vi "simple data display custom vi.vi"(9 "customQueue":refnum<queue>, 11 "parentQueue":refnum<queue>) -> ()   [LabVIEW 2018]
uses:
  custom sub vis/plotControl.ctl
  customViData.ctl
panel:
  out "mainMessage":string caption="Message received from Main VI"
  in  "plotType":bool
  in  "plotControl":T1[](array[typedef])=[{"channel"="time", "X"=TRUE, "Y"=FALSE, "Y2"=FALSE}]
  out "dataTable":string[][](table)
  out "XY Graph":cluster{"New data":dbl[], "New data":dbl[]}[](graph)
  in  "really stop":bool
  in  "quit":bool
  out "ballValve":dbl caption="ball Valve"
  out "butterflyValve":dbl caption="butterfly Valve"
  out "speed":dbl caption="compressor Speed"
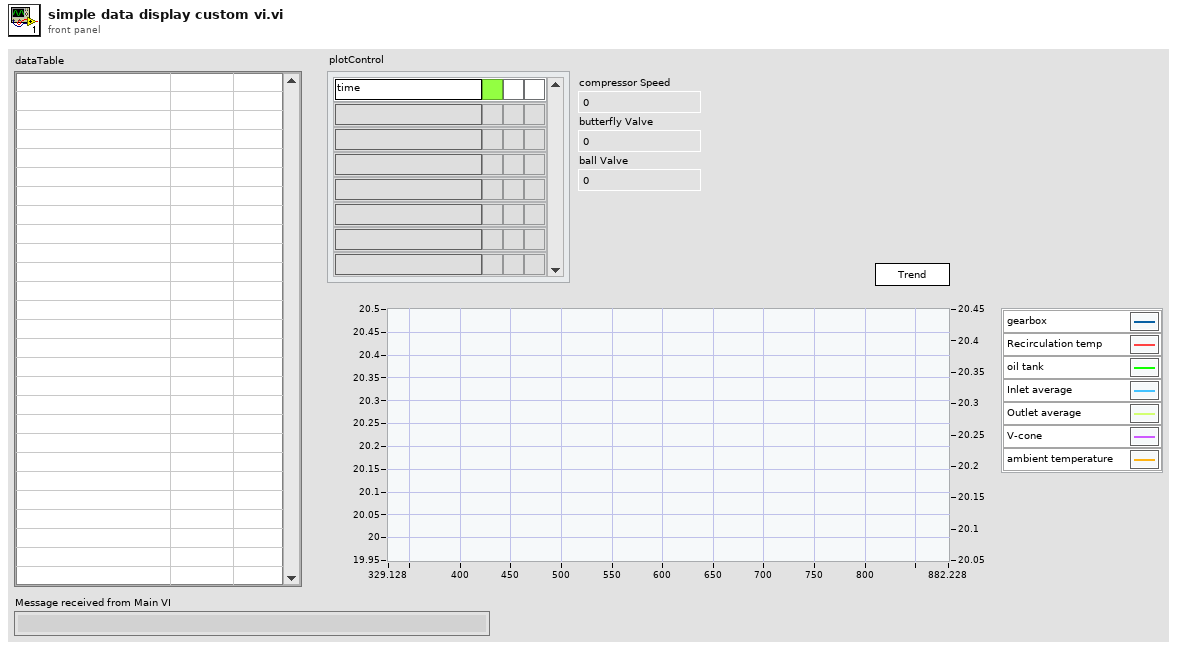
[diagram p1: front panel]
types:
  T1 = typedef "plotControl.ctl" = cluster{"channel":string, "X":bool, "Y":bool, "Y2":bool}
  T2 = typedef "customViData.ctl" = cluster{"rigChannels":string[], "rigUnits":string[], "logging":bool, "plot":cluster{"X":u16[], "Y":u16[], "Y2":u16[]}, "updatePlot":bool, "chartRef":refnum<vi>, "livePlot":bool, "history":dbl[][], "channelCount":i32, "trendIndex":i32}
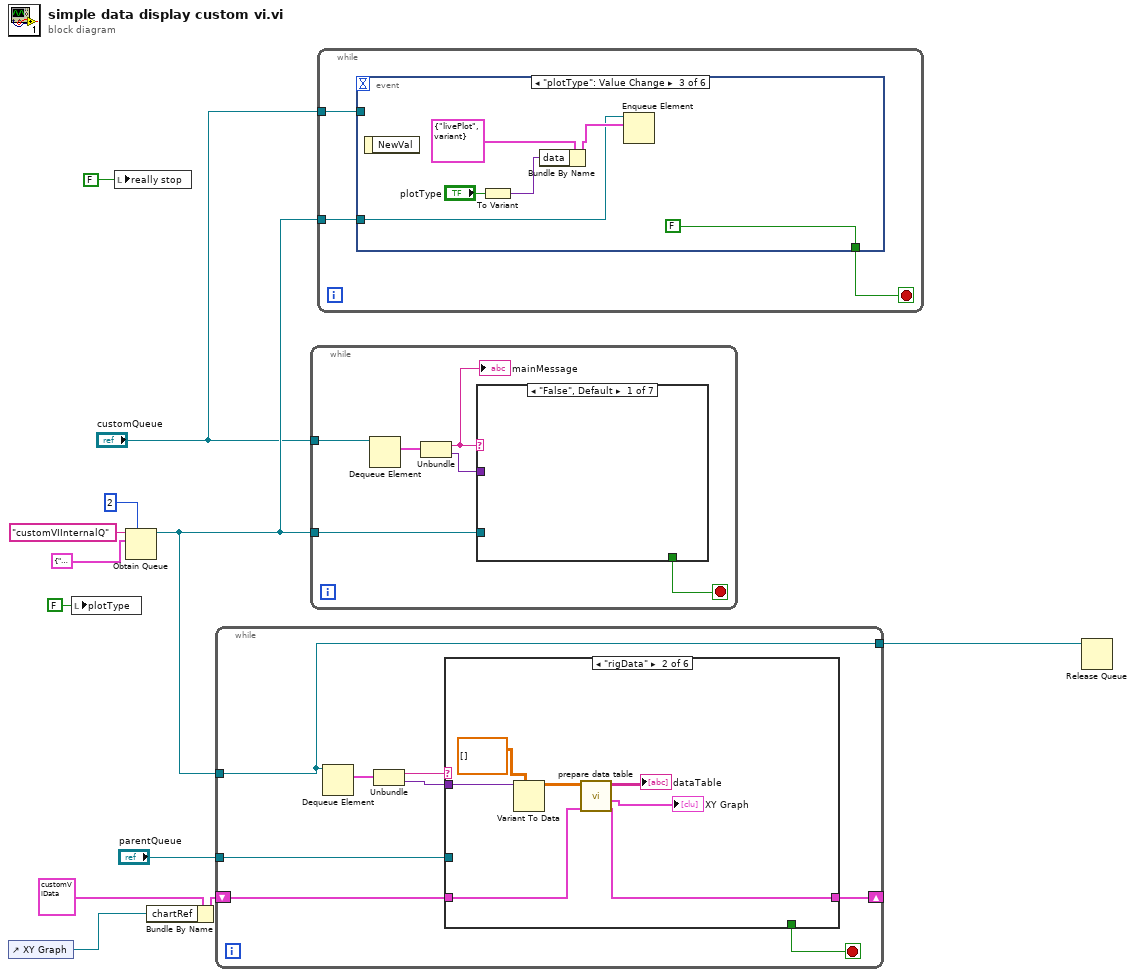
[diagram p0: block diagram]
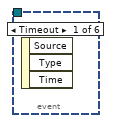
[diagram p2: hidden frame]
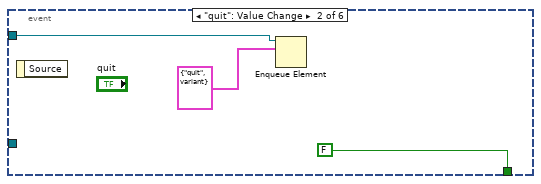
[diagram p3: hidden frame]
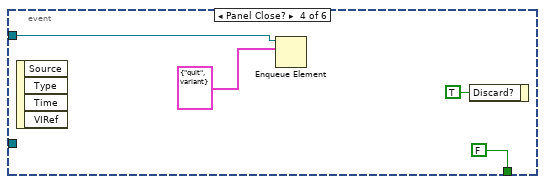
[diagram p4: hidden frame]
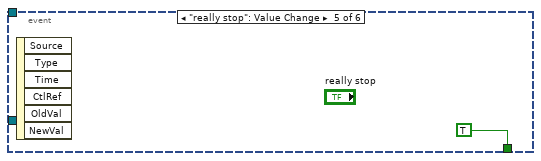
[diagram p5: hidden frame]
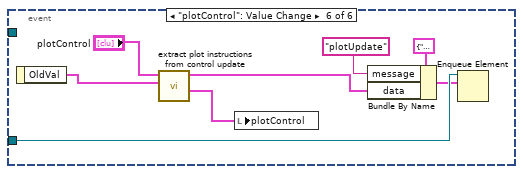
[diagram p6: hidden frame]
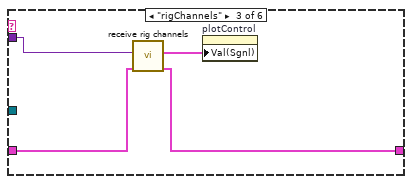
[diagram p8: hidden frame]
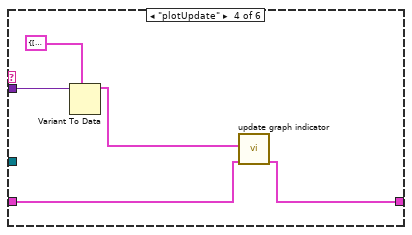
[diagram p9: hidden frame]
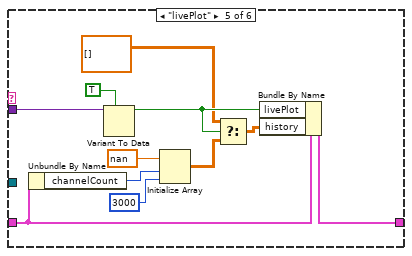
[diagram p10: hidden frame]
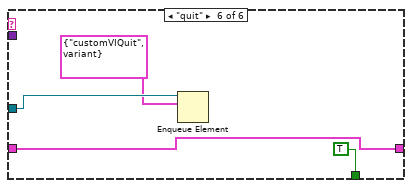
[diagram p11: hidden frame]
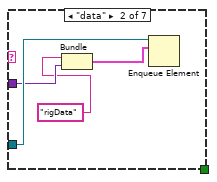
[diagram p12: hidden frame]
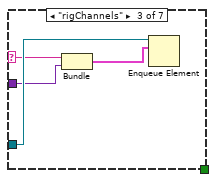
[diagram p13: hidden frame]
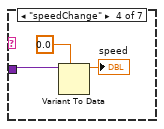
[diagram p14: hidden frame]
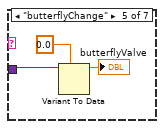
[diagram p15: hidden frame]
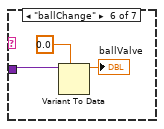
[diagram p16: hidden frame]
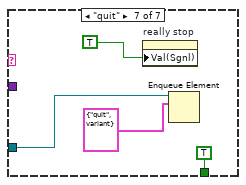
[diagram p17: hidden frame]
diagram:
  n1 = control-ref of="XY Graph"() -> (w2:refnum<vi>)
  n2 = local write "plotType"(FALSE ("plotType")) -> ()
  n3 = local write "really stop"(FALSE) -> ()
  n4 = Obtain Queue(max queue size (-1, unlimited)=2, name (unnamed)="customVIInternalQ", element data type=cluster{"message":string, "data":variant} {"message"="", "data"=variant} ("element")) -> (queue out=w9:refnum<queue>)  [unwired: 2 in, 2 out]
  n5 = Bundle By Name(cluster=T2 {"rigChannels"=[], "rigUnits"=[], "logging"=FALSE, "plot"={"X"=[], "Y"=[], "Y2"=[]}, "updatePlot"=FALSE, "chartRef"=refnum, "livePlot"=FALSE, "history"=[], "channelCount"=0, "trendIndex"=0}, "chartRef"=w2) -> (w3:T2)
  n6 = while {
    tunnel: w9 -> [w15]
    tunnel: "parentQueue" -> [w17]
    tunnel: [w15] -> w7
    shift-right: [w14] -> _
    shift-left: w3 -> [w13]
    stop <- w16 stop-if-true
    n7 = Dequeue Element(queue=w15) -> (element=w20:cluster{"message":string, "data":variant})  [unwired: 2 in, 3 out]
    n8 = Unbundle(w20) -> ("message"=w19:string, "data"=w18:variant)
    n9 = case shown="\"rigData\"" w19 {
      tunnel: w18 -> [_ w28 w32 w37 w47 _]
      tunnel: w17 -> [_ _ _ _ _ w52]
      tunnel: [_ _ _ _ _ TRUE] -> w16
      tunnel: [w21 w23 w30 w34 w48 w49] -> w14
      tunnel: w13 -> [w21 w26 w31 w35 w44 w49]
      frame "", Default {
      }
      frame "rigData" {
        n10 = Variant To Data(type=dbl[][] [], Variant=w28) -> (data=w25:dbl[][])  [unwired: 1 in, 1 out]
        n11 = call "prepare data table.vi"("customViData"=w26, "New data"=w25) -> ("customViData out"=w23:T2, "plot data"=→"XY Graph":cluster{"New data":dbl[], "New data":dbl[]}[], "dataTable"=→"dataTable":string[][])  [unwired: 6 in, 1 out]
      }
      frame "rigChannels" {
        n12 = call "receive rig channels.vi"("customViData in"=w31, "data"=w32) -> ("customViData out"=w30:T2, "updated plotControl"=w29:T1[])  [unwired: 8 in]
        n13 = property on="plotControl" class="Arr (strict)"("Val(Sgnl)"=w29) -> ()  [unwired: 2 in, 2 out]
      }
      frame "plotUpdate" {
        n14 = Variant To Data(type=cluster{"X":u16[], "Y":u16[], "Y2":u16[]} {"X"=[], "Y"=[], "Y2"=[]} ("plot"), Variant=w37) -> (data=w36:cluster{"X":u16[], "Y":u16[], "Y2":u16[]})  [unwired: 1 in, 1 out]
        n15 = call "update graph indicator.vi"("customViData in"=w35, "plot"=w36) -> ("customViData out"=w34:T2)  [unwired: 9 in]
      }
      frame "livePlot" {
        n16 = Unbundle By Name(w44) -> ("channelCount"=w43:i32)
        n17 = Variant To Data(type=TRUE, Variant=w47) -> (data=w41:bool)  [unwired: 1 in, 1 out]
        n18 = Initialize Array(nan ("element"), w43, 3000 ("dimension size")) -> (w39:dbl[][])
        n19 = Select(t=dbl[][] [] ("history"), s=w41, f=w39) -> (s? t:f=w38:dbl[][])
        n20 = Bundle By Name(cluster=w44, "livePlot"=w41, "history"=w38) -> (w48:T2)
      }
      frame "quit" {
        n21 = Enqueue Element(queue=w52, element=cluster{"message":string, "data":variant} {"message"="customVIQuit", "data"=variant}) -> ()  [unwired: 2 in, 3 out]
      }
    }
  }
  n22 = while {
    tunnel: "customQueue" -> [w58]
    tunnel: w9 -> [w55]
    stop <- w54 stop-if-true
    n23 = Dequeue Element(queue=w58) -> (element=w57:cluster{"message":string, "data":variant})  [unwired: 2 in, 3 out]
    n24 = Unbundle(w57) -> ("message"=w53:string, "data"=w56:variant)
    "mainMessage" <- w53
    n25 = case shown="\"False\", Default" w53 {
      selector: w53 -> [_ _ w63 _ _ _ _]
      tunnel: w56 -> [_ w61 w65 w69 w72 w75 _]
      tunnel: w55 -> [_ w62 w66 _ _ _ w78]
      tunnel: [_ _ _ _ _ _ TRUE] -> w54
      frame "False", Default {
      }
      frame "data" {
        n26 = Bundle("rigData", "data"=w61) -> (w60:cluster{string, "data":variant})  [unwired: 1 in]
        n27 = Enqueue Element(queue=w62, element=w60) -> ()  [unwired: 2 in, 3 out]
      }
      frame "rigChannels" {
        n28 = Bundle(w63, "data"=w65) -> (w64:cluster{string, "data":variant})  [unwired: 1 in]
        n29 = Enqueue Element(queue=w66, element=w64) -> ()  [unwired: 2 in, 3 out]
      }
      frame "speedChange" {
        n30 = Variant To Data(type=0.0 ("y"), Variant=w69) -> (data=→"speed":dbl)  [unwired: 1 in, 1 out]
      }
      frame "butterflyChange" {
        n31 = Variant To Data(type=0.0 ("y"), Variant=w72) -> (data=→"butterflyValve":dbl)  [unwired: 1 in, 1 out]
      }
      frame "ballChange" {
        n32 = Variant To Data(type=0.0 ("y"), Variant=w75) -> (data=→"ballValve":dbl)  [unwired: 1 in, 1 out]
      }
      frame "quit" {
        n33 = property on="really stop" class="Bool (strict)"("Val(Sgnl)"=TRUE) -> ()  [unwired: 2 in, 2 out]
        n34 = Enqueue Element(queue=w78, element=cluster{"message":string, "data":variant} {"message"="quit", "data"=variant}) -> ()  [unwired: 2 in, 3 out]
      }
    }
  }
  n35 = while {
    tunnel: w9 -> [w82]
    tunnel: "customQueue" -> [w80]
    stop <- w81 stop-if-true
    n36 = event shown="[2] \"plotType\": Value Change" {
      selector: _ -> [_ _ _ _ _ _]
      dyn-events: _ -> [_ _ _ _ _ _]
      timeout: _ -> [_ _ _ _ _ _]
      tunnel: w82 -> [_ _ w86 _ _ w103]
      tunnel: [_ FALSE FALSE FALSE TRUE _] -> w81
      tunnel: w80 -> [_ w83 _ w93 _ _]
      event Timeout {
        n37 = event-data() -> ()  [unwired: 1 in, 3 out]
      }
      event "quit": Value Change {
        n38 = event-data() -> ()  [unwired: 1 in, 1 out]
        n39 = Enqueue Element(queue=w83, element=cluster{"message":string, "data":variant} {"message"="quit", "data"=variant}) -> ()  [unwired: 2 in, 3 out]
      }
      event "plotType": Value Change {
        n40 = event-data() -> ()  [unwired: 1 in, 1 out]
        n41 = To Variant(anything="plotType") -> (Variant=w87:variant)
        n42 = Bundle By Name(cluster=cluster{"message":string, "data":variant} {"message"="livePlot", "data"=variant} ("element"), "data"=w87) -> (w89:cluster{"message":string, "data":variant})
        n43 = Enqueue Element(queue=w86, element=w89) -> ()  [unwired: 2 in, 3 out]
      }
      event Panel Close? {
        n44 = event-data() -> ()  [unwired: 1 in, 4 out]
        n45 = Enqueue Element(queue=w93, element=cluster{"message":string, "data":variant} {"message"="quit", "data"=variant}) -> ()  [unwired: 2 in, 3 out]
        n46 = event-data("Discard?"=TRUE) -> ()  [unwired: 1 in, 1 out]
      }
      event "really stop": Value Change {
        n47 = event-data() -> ()  [unwired: 1 in, 6 out]
      }
      event "plotControl": Value Change {
        n48 = event-data() -> ("OldVal"=w100:T1[])  [unwired: 1 in]
        n49 = call "extract plot instructions from control update.vi"("OldVal"=w100, "Plot Control"="plotControl") -> ("correctControl"=w98:T1[], "plotUpdate"=w99:cluster{"X":u16[], "Y":u16[], "Y2":u16[]})  [unwired: 8 in]
        n50 = local write "plotControl"(w98) -> ()
        n51 = Bundle By Name(cluster=cluster{"message":string, "data":variant} {"message"="", "data"=variant} ("element"), "message"="plotUpdate", "data"=w99) -> (w102:cluster{"message":string, "data":variant})
        n52 = Enqueue Element(queue=w103, element=w102) -> ()  [unwired: 2 in, 3 out]
      }
    }
  }
  n53 = Release Queue(queue=w7) -> ()  [unwired: 2 in, 3 out]
